vi "RT_Main.vi"() -> ()   [LabVIEW 2018]
uses:
  <vilib>/NI/STM/SubVIs/MetaDataElement.ctl
  RT_Listener_states.ctl
  RT_Counter_FGV_States.ctl
  RT_Comm_Manager_Message.ctl
  RT_Comm_Manager_States.ctl
  <vilib>/NI/STM/TCP/TCP Connection Info.ctl
  <vilib>/NI/STM/Connection Manager/TCP/TCP Connection Method.ctl
  <vilib>/NI/STM/TCP/TCP Write Options.ctl
  <vilib>/NI/STM/TCP/TCP Read Options.ctl
  <vilib>/NI/STM/TCP/Get Connection Reference (TCP).vi
  <vilib>/NI/STM/TCP/Read Meta Data (TCP Ref).vi
  <vilib>/NI/STM/SubVIs/Generate STM Error.vi
  <vilib>/NI/STM/TCP/Read Meta Data (TCP Clst).vi
  <vilib>/NI/STM/TCP/Read Message (TCP).vi
  <vilib>/NI/STM/TCP/Write Message (TCP).vi
  <vilib>/NI/STM/NI STM.lvlib
panel:
  out "Sensor not connected":bool
  out "meta data":T1[](array[typedef])
  in  "Max connections":i32=10
  out "Number of connections":i32
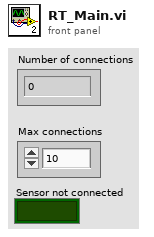
[diagram p1: front panel]
types:
  T1 = typedef "NI STM.lvlib/MetaDataElement.ctl" = string
  T2 = typedef "NI STM.lvlib/TCP Connection Info.ctl" = cluster{"connection ID":refnum<k5>, "meta data":T1[]}
  T3 = typedef "RT_Comm_Manager_Message.ctl" = cluster{"RT Comm Manager States":T4, "Data":variant}
  T4 = typedef "RT_Comm_Manager_States.ctl" = enum16{"Meas finished", "New connection", "Exit"}
  T5 = typedef "RT_Counter_FGV_States.ctl" = enum16{"Init", "Increase", "Decrease", "Get"}
  T6 = typedef "RT_Listener_states.ctl" = enum16{"Idle", "Listen", "Wait", "Exit"}
  T7 = typedef "NI STM.lvlib/TCP Connection Manager Reference.ctl" = refnum<data-value>
  T8 = typedef "NI STM.lvlib/TCP Read Options.ctl" = cluster{"ignore timeout error":bool, "timeout ms (1000)":i32}
  T9 = typedef "NI STM.lvlib/TCP Write Options.ctl" = cluster{"ignore timeout error":bool, "timeout ms (1000)":i32}
  T10 = typedef "NI STM.lvlib/TCP Connection Method.ctl" = enum16{"Initialize", "Add Connection", "Set Properties", "Get Connection(s)", "Remove Connection", "Remove All Connections", "Get Connection Count"}
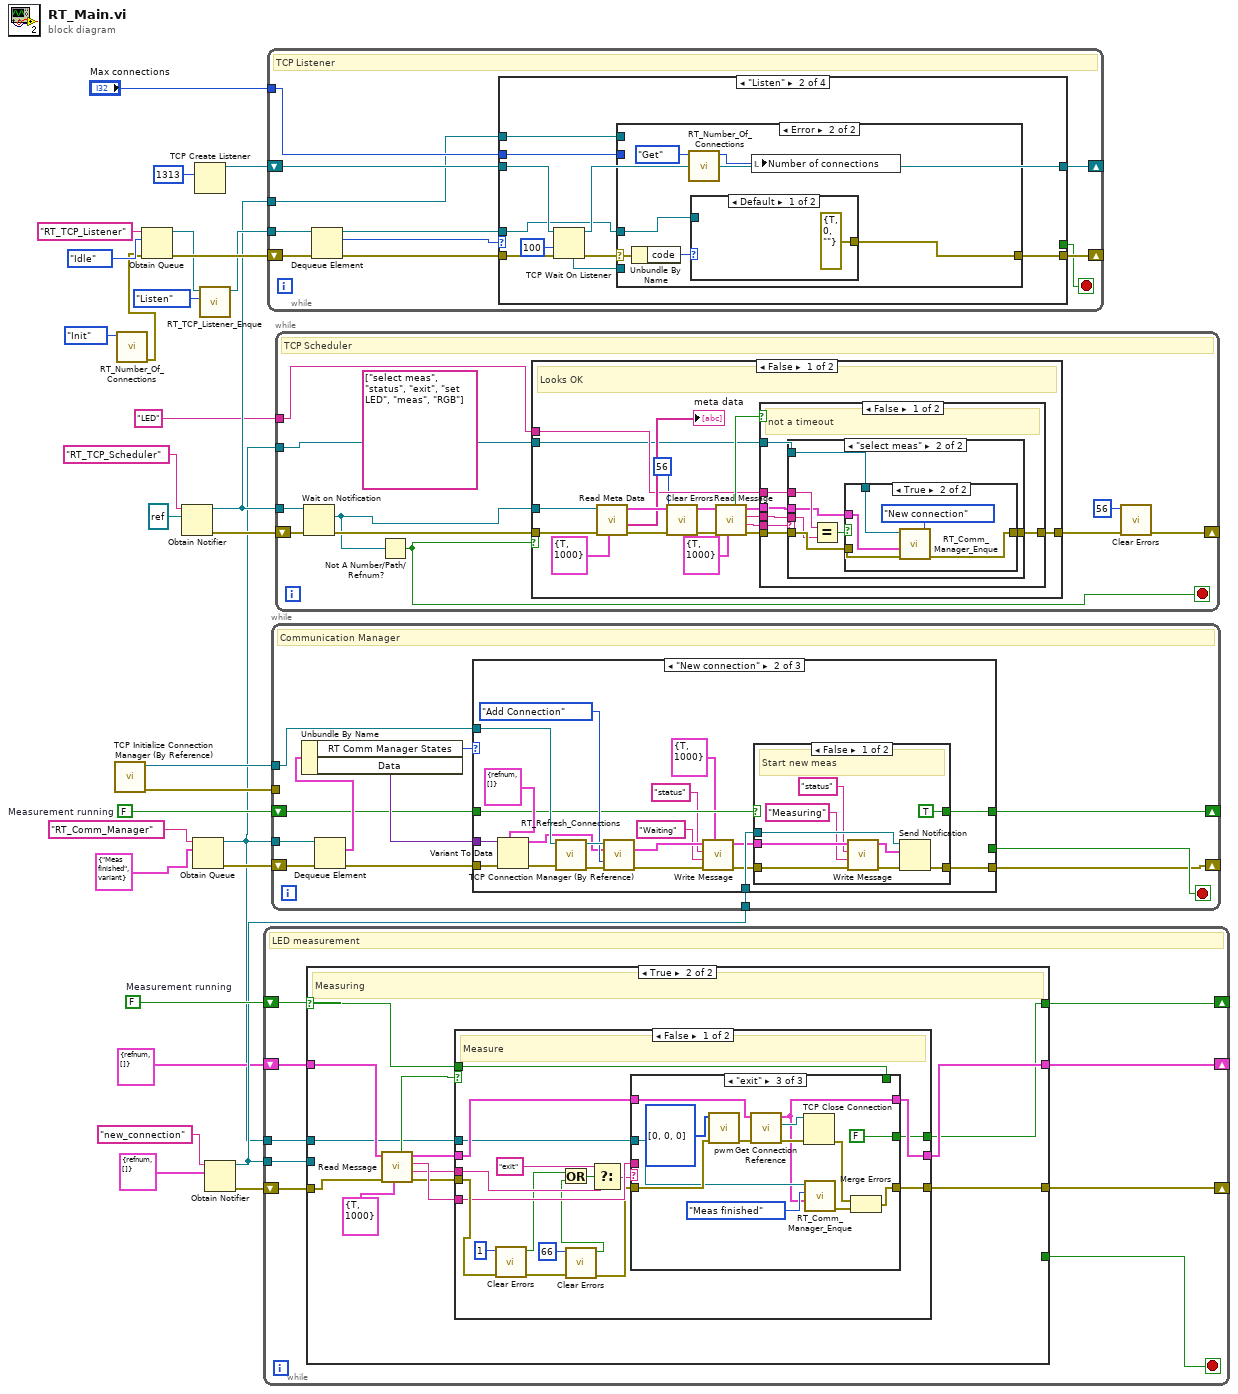
[diagram p0: block diagram]
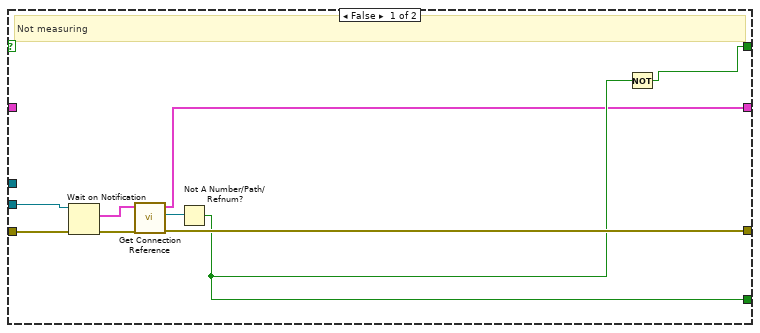
[diagram p2: hidden frame]
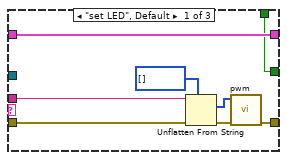
[diagram p3: hidden frame]
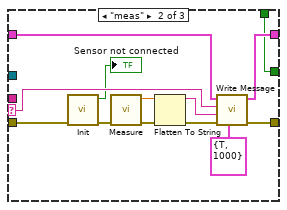
[diagram p4: hidden frame]
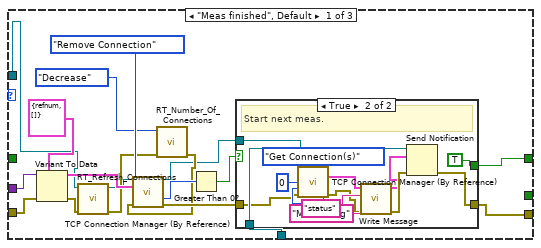
[diagram p6: hidden frame]
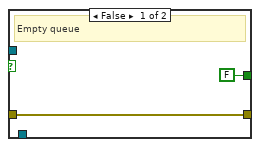
[diagram p7: hidden frame]
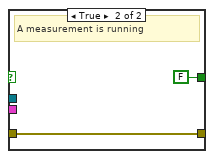
[diagram p8: hidden frame]
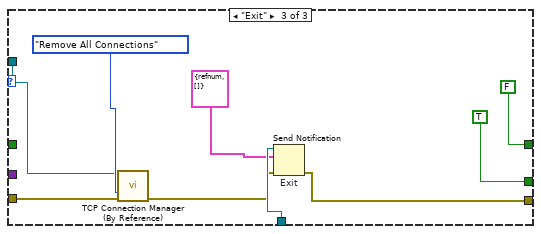
[diagram p9: hidden frame]
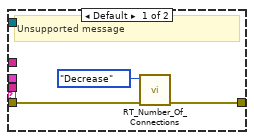
[diagram p10: hidden frame]
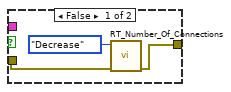
[diagram p11: hidden frame]
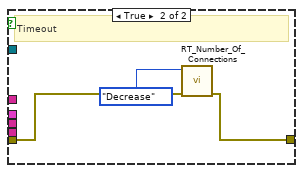
[diagram p12: hidden frame]
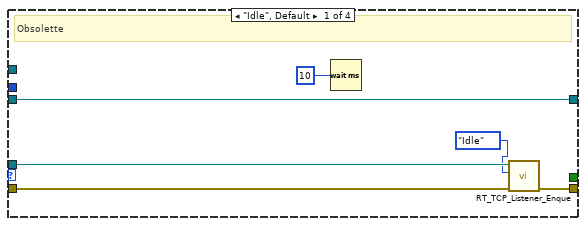
[diagram p14: hidden frame]
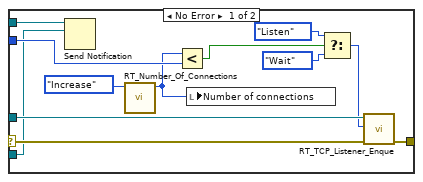
[diagram p15: hidden frame]
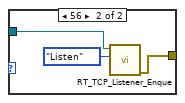
[diagram p16: hidden frame]
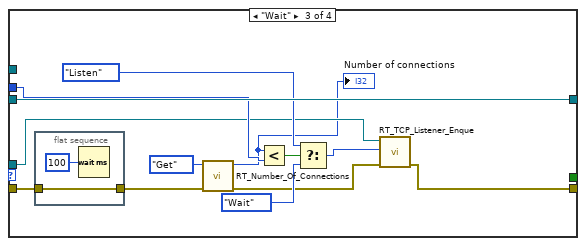
[diagram p17: hidden frame]
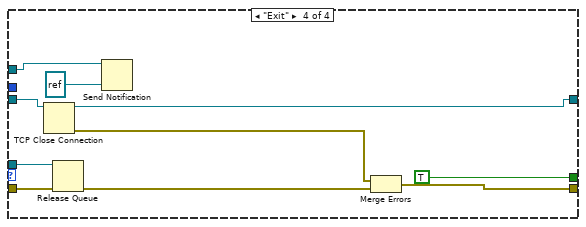
[diagram p18: hidden frame]
diagram:
  w7 = FALSE  # Measurement running
  w8 = FALSE  # Measurement running
  n1 = call <vilib>:"TCP Initialize Connection Manager (By Reference).vi"() -> ("error out"=w14:errorcluster, "connection manager ref out"=w13:T7)  [unwired: 10 in]
  n2 = call "RT_Number_Of_Connections.vi"("Counter_FGV_States"=RT_Counter_FGV_States."Init") -> ("Error Out"=w20:errorcluster)  [unwired: 9 in, 1 out]
  n3 = Obtain Queue(name (unnamed)="RT_TCP_Listener", element data type=RT_Listener_states."Idle" ("Listener States"), error in (no error)=w20) -> (queue out=w24:refnum<queue>, error out=w27:errorcluster)  [unwired: 2 in, 1 out]
  n4 = Obtain Notifier(name (unnamed)="RT_TCP_Scheduler", notification data type=refnum<k5> refnum ("connection ID")) -> (notifier out=w16:refnum<notifier>, error out=w15:errorcluster)  [unwired: 2 in, 1 out]
  n5 = Obtain Queue(name (unnamed)="RT_Comm_Manager", element data type=T3 {"RT Comm Manager States"=enum."Meas finished", "Data"=variant} ("Comm Manager Message")) -> (queue out=w1:refnum<queue>, error out=w9:errorcluster)  [unwired: 3 in, 1 out]
  n6 = TCP Create Listener(10:u16 1313 ("port")) -> (3:w25:refnum<k5>)  [unwired: 4 in, 2 out]
  n7 = call "RT_TCP_Listener_Enque.vi"("Listener States"=RT_Listener_states."Listen", "Queue In"=w24) -> ("Queue Out"=w23:refnum<queue>)  [unwired: 8 in, 1 out]
  n8 = Obtain Notifier(name (unnamed)="new_connection", notification data type=T2 {"connection ID"=refnum, "meta data"=[]} ("connection info out")) -> (notifier out=w3:refnum<notifier>, error out=w4:errorcluster)  [unwired: 2 in, 1 out]
  n9 = while {
    shift-right: [w37] -> _
    shift-left: w7 -> [w38]
    tunnel: w3 -> [w36]
    shift-right: [w33] -> _
    shift-left: w4 -> [w35]
    shift-right: [w32] -> _
    shift-left: T2 {"connection ID"=refnum, "meta data"=[]} ("connection info out") -> [w31]
    tunnel: w1 -> [w30]
    stop <- w34 stop-if-true
    # "LED measurement"
    n10 = case shown="True" w38 {
      selector: w38 -> [_ w48]
      tunnel: [w40 w49] -> w37
      tunnel: w36 -> [w47 _]
      tunnel: w35 -> [w46 w58]
      tunnel: [w41 _] -> w34
      tunnel: [w42 w60] -> w33
      tunnel: [w39 w54] -> w32
      tunnel: w31 -> [_ w57]
      tunnel: w30 -> [_ w51]
      frame False {
        # "Not measuring"
        n11 = Wait on Notification(notifier=w47, error in (no error)=w46) -> (notification=w44:T2, error out=w45:errorcluster)  [unwired: 2 in, 2 out]
        n12 = call-poly <vilib>:"Get Connection Reference.vi"("error in"=w45, "connection info in"=w44) -> ("error out"=w42:errorcluster, "connection ID out"=w43:refnum<k5>, "connection info out"=w39:T2)  [unwired: 7 in]
        n13 = Not A Number/Path/Refnum?(number/path/refnum=w43) -> (NaN/Path/Refnum?=w41:bool)
        n14 = Not(x=w41) -> (.not. x?=w40:bool)
      }
      frame True {
        # "Measuring"
        n15 = call-poly <vilib>:"Read Message.vi"("options"=T8 {"ignore timeout error"=TRUE, "timeout ms (1000)"=1000}, "error in"=w58, "connection info in"=w57) -> ("error out"=w50:errorcluster, "name"=w52:T1, "data string"=w53:string, "connection info out"=w55:T2, "timed out?"=w56:bool)  [unwired: 3 in, 1 out]
        n16 = case shown="False" w56 {
          tunnel: [w78 w114] -> w60
          tunnel: w50 -> [w77 w114]
          tunnel: w55 -> [w75 w115]
          tunnel: [w76 w115] -> w54
          tunnel: w53 -> [w74 _]
          tunnel: w52 -> [w71 _]
          tunnel: w51 -> [w73 _]
          tunnel: [w68 w113] -> w49
          tunnel: w48 -> [w67 w113]
          frame False {
            # "Measure"
            n17 = call <vilib>:"Clear Errors.vi"("error in (no error)"=w77, "specific error code to clear (0: all)"=1) -> ("error out"=w64:errorcluster, "specific error cleared?"=w70:bool)  [unwired: 4 in]
            n18 = call <vilib>:"Clear Errors.vi"("error in (no error)"=w64, "specific error code to clear (0: all)"=66) -> ("error out"=w63:errorcluster, "specific error cleared?"=w61:bool)  [unwired: 4 in]
            n19 = Or(x=w70, y=w61) -> (x .or. y?=w62:bool)
            n20 = Select(t=T1 "exit", s=w62, f=w71) -> (s? t:f=w72:T1)
            n21 = case shown="\"exit\"" w72 {
              selector: w72 -> [_ w96 _]
              tunnel: [w81 w98 w101] -> w76
              tunnel: [w83 w99 w104] -> w78
              tunnel: w63 -> [w82 w89 w108]
              tunnel: w75 -> [w81 w88 w107]
              tunnel: w74 -> [w80 _ _]
              tunnel: w73 -> [_ _ w103]
              tunnel: [w79 w87 FALSE] -> w68
              tunnel: w67 -> [w79 w87 _]
              frame "set LED", Default {
                n22 = Unflatten From String(type=u8[] [], binary string=w80, error in (no error)=w82) -> (value=w85:u8[], error out=w86:errorcluster)  [unwired: 2 in, 1 out]
                n23 = call "pwm.vi"("Error In"=w86, "PWMs"=w85) -> ("Error Out"=w83:errorcluster)  [unwired: 9 in]
              }
              frame "meas" {
                n24 = call "Init.vi"("Error In"=w89) -> ("Error Out"=w91:errorcluster, "Not connected"=→"Sensor not connected":bool)  [unwired: 9 in]
                n25 = call "Measure.vi"("Error In"=w91) -> ("Error Out"=w93:errorcluster, "Luminosity"=w92:dbl)  [unwired: 9 in]
                n26 = Flatten To String(anything=w92, error in (no error)=w93) -> (data string=w94:string, error out=w95:errorcluster)  [unwired: 2 in, 1 out]
                n27 = call-poly <vilib>:"Write Message.vi"("options"=T9 {"ignore timeout error"=TRUE, "timeout ms (1000)"=1000}, "error in"=w95, "data"=w94, "name"=w96, "connection info in"=w88) -> ("error out"=w99:errorcluster, "connection info out"=w98:T2)  [unwired: 5 in]
              }
              frame "exit" {
                n28 = call "pwm.vi"("Error In"=w108, "PWMs"=u8[] [0, 0, 0]) -> ("Error Out"=w110:errorcluster)  [unwired: 9 in]
                n29 = call-poly <vilib>:"Get Connection Reference.vi"("error in"=w110, "connection info in"=w107) -> ("error out"=w112:errorcluster, "connection ID out"=w111:refnum<k5>, "connection info out"=w101:T2)  [unwired: 7 in]
                n30 = TCP Close Connection(connection ID=w111, error in (no error)=w112) -> (error out=w105:errorcluster)  [unwired: 1 in, 1 out]
                n31 = call "RT_Comm_Manager_Enque.vi"("Data"=w101, "Next State"=RT_Comm_Manager_States."Meas finished", "Queue In"=w103) -> ("Error Out"=w106:errorcluster)  [unwired: 7 in, 1 out]
                n32 = Merge Errors(w105, w106) -> (w104:errorcluster)
              }
            }
          }
          frame True {
            # "Timeout"
          }
        }
      }
    }
  }
  n33 = while {
    tunnel: w23 -> [w126]
    shift-right: [w121] -> _
    shift-left: w27 -> [w125]
    shift-right: [w118] -> _
    shift-left: w25 -> [w119]
    tunnel: "Max connections" -> [w117]
    tunnel: w16 -> [w116]
    stop <- w120 stop-if-true
    # "TCP Listener"
    n34 = Dequeue Element(queue=w126, error in (no error)=w125) -> (queue out=w122:refnum<queue>, element=w123:T6, error out=w124:errorcluster)  [unwired: 1 in, 1 out]
    n35 = case shown="\"Listen\"" w123 {
      tunnel: w124 -> [w131 w142 w174 w189]
      tunnel: w122 -> [w129 w138 w166 w186]
      tunnel: [w130 w137 w168 w184] -> w121
      tunnel: [_ _ _ TRUE] -> w120
      tunnel: w119 -> [w132 w141 w177 w185]
      tunnel: [w132 w140 w177 w182] -> w118
      tunnel: w117 -> [_ w134 w173 _]
      tunnel: w116 -> [_ w133 _ w181]
      frame "Idle", Default {
        # "Obsolette"
        n36 = Wait (ms)(milliseconds to wait=u32 10) -> ()  [unwired: 1 out]
        n37 = call "RT_TCP_Listener_Enque.vi"("Error In"=w131, "Listener States"=RT_Listener_states."Idle", "Queue In"=w129) -> ("Error Out"=w130:errorcluster)  [unwired: 7 in, 1 out]
      }
      frame "Listen" {
        n38 = TCP Wait On Listener(8:w142, 9:100 ("timeout ms (wait forever: -1)"), 11:w141) -> (0:w136:errorcluster, 3:w140:refnum<k5>, 4:w135:refnum<k5>)  [unwired: 1 in, 2 out]
        n39 = case shown="Error" w136 {
          selector: w136 -> [w152 w160]
          tunnel: w138 -> [w154 w158]
          tunnel: [w153 w157] -> w137
          tunnel: w135 -> [w144 _]
          tunnel: w134 -> [w150 _]
          tunnel: w133 -> [w145 _]
          frame No Error {
            n40 = Send Notification(notification=w144, notifier=w145) -> ()  [unwired: 1 in, 2 out]
            n41 = call "RT_Number_Of_Connections.vi"("Counter_FGV_States"=RT_Counter_FGV_States."Increase") -> ("Number of connections"=w143:i32)  [unwired: 9 in, 1 out]
            n42 = Less?(x=w143, y=w150) -> (x < y?=w149:bool)
            n43 = local write "Number of connections"(w143) -> ()
            n44 = Select(t=RT_Listener_states."Listen" ("Listener States"), s=w149, f=RT_Listener_states."Wait") -> (s? t:f=w146:T6)
            n45 = call "RT_TCP_Listener_Enque.vi"("Error In"=w152, "Listener States"=w146, "Queue In"=w154) -> ("Error Out"=w153:errorcluster)  [unwired: 7 in, 1 out]
          }
          frame Error {
            n46 = Unbundle By Name(w160) -> ("code"=w159:i32)
            n47 = call "RT_Number_Of_Connections.vi"("Counter_FGV_States"=RT_Counter_FGV_States."Get") -> ("Number of connections"=w155:i32)  [unwired: 9 in, 1 out]
            n48 = case shown="Default" w159 {
              tunnel: w158 -> [_ w164]
              tunnel: [errorcluster {"status"=TRUE, "code"=0, "source"=""} ("Error Out") w162] -> w157
              frame Default {
              }
              frame 56 {
                n49 = call "RT_TCP_Listener_Enque.vi"("Listener States"=RT_Listener_states."Listen", "Queue In"=w164) -> ("Error Out"=w162:errorcluster)  [unwired: 8 in, 1 out]
              }
            }
            n50 = local write "Number of connections"(w155) -> ()
          }
        }
      }
      frame "Wait" {
        n51 = flat-sequence {
          tunnel: [w178] -> w175
          tunnel: w174 -> [w178]
          frame #0 {
            n52 = Wait (ms)(milliseconds to wait=u32 100) -> ()  [unwired: 1 out]
          }
        }
        n53 = call "RT_Number_Of_Connections.vi"("Error In"=w175, "Counter_FGV_States"=RT_Counter_FGV_States."Get") -> ("Error Out"=w169:errorcluster, "Number of connections"=w165:i32)  [unwired: 8 in]
        "Number of connections" <- w165
        n54 = Less?(x=w165, y=w173) -> (x < y?=w172:bool)
        n55 = Select(t=RT_Listener_states."Listen" ("Listener States"), s=w172, f=RT_Listener_states."Wait" ("Listener States")) -> (s? t:f=w167:T6)
        n56 = call "RT_TCP_Listener_Enque.vi"("Error In"=w169, "Listener States"=w167, "Queue In"=w166) -> ("Error Out"=w168:errorcluster)  [unwired: 7 in, 1 out]
      }
      frame "Exit" {
        n57 = TCP Close Connection(connection ID=w185) -> (connection ID out=w182:refnum<k5>, error out=w183:errorcluster)  [unwired: 2 in]
        n58 = Release Queue(queue=w186, error in (no error)=w189) -> (error out=w188:errorcluster)  [unwired: 1 in, 2 out]
        n59 = Send Notification(notification=refnum<k5> refnum ("connection ID"), notifier=w181) -> ()  [unwired: 1 in, 2 out]
        n60 = Merge Errors(w183, w188) -> (w184:errorcluster)
      }
    }
  }
  n61 = while {
    tunnel: w14 -> [_]
    tunnel: w13 -> [w195]
    tunnel: w1 -> [w201]
    shift-right: [w193] -> _
    shift-left: w9 -> [w200]
    shift-right: [w191] -> _
    shift-left: w8 -> [w192]
    tunnel: w3 -> [w190]
    stop <- w194 stop-if-true
    # "Communication Manager"
    n62 = Dequeue Element(queue=w201, error in (no error)=w200) -> (element=w199:T3, error out=w197:errorcluster)  [unwired: 1 in, 2 out]
    n63 = Unbundle By Name(w199) -> ("RT Comm Manager States"=w198:T4, "Data"=w196:variant)
    n64 = case shown="\"New connection\"" w198 {
      tunnel: w197 -> [w217 w254 w274]
      tunnel: w196 -> [w215 w253 _]
      tunnel: w195 -> [w207 w250 w270]
      tunnel: [w209 w244 w266] -> w193
      tunnel: [_ _ TRUE] -> w194
      tunnel: w192 -> [_ w245 _]
      tunnel: [w210 w243 FALSE] -> w191
      tunnel: w190 -> [w208 w242 w269]
      frame "Meas finished", Default {
        n65 = Variant To Data(error in=w217, type=T2 {"connection ID"=refnum, "meta data"=[]} ("connection info out"), Variant=w215) -> (data=w214:T2, error out=w216:errorcluster)
        n66 = call "RT_Refresh_Connections.vi"("Error In"=w216, "connection manager ref in"=w207) -> ("Error Out"=w204:errorcluster, "connection manager ref out"=w206:T7)  [unwired: 8 in]
        n67 = call "RT_Number_Of_Connections.vi"("Error In"=w204, "Counter_FGV_States"=RT_Counter_FGV_States."Decrease") -> ("Error Out"=w203:errorcluster)  [unwired: 8 in, 1 out]
        n68 = call <vilib>:"TCP Connection Manager (By Reference).vi"("connection manager ref in"=w206, "connection in"=w214, "method"=TCP_Connection_Method."Remove Connection", "error in"=w203) -> ("connection manager ref out"=w202:T7, "number of connections"=w213:i32, "error out"=w212:errorcluster)  [unwired: 5 in, 4 out]
        n69 = Greater Than 0?(x=w213) -> (x > 0?=w211:bool)
        n70 = case shown="True" w211 {
          tunnel: w212 -> [w221 w228]
          tunnel: [FALSE TRUE] -> w210
          tunnel: [w221 w232] -> w209
          tunnel: w208 -> [_ w233]
          tunnel: w202 -> [_ w229]
          frame False {
            # "Empty queue"
          }
          frame True {
            # "Start next meas."
            n71 = call <vilib>:"TCP Connection Manager (By Reference).vi"("connection manager ref in"=w229, "index"=0, "method"=TCP_Connection_Method."Get Connection(s)", "error in"=w228) -> ("connection out"=w227:T2, "error out"=w223:errorcluster)  [unwired: 5 in, 5 out]
            n72 = call-poly <vilib>:"Write Message.vi"("error in"=w223, "data"="Measuring", "name"="status", "connection info in"=w227) -> ("error out"=w224:errorcluster, "connection info out"=w222:T2)  [unwired: 6 in]
            n73 = Send Notification(notification=w222, notifier=w233, error in (no error)=w224) -> (error out=w232:errorcluster)  [unwired: 1 out]
          }
        }
      }
      frame "New connection" {
        n74 = Variant To Data(error in=w254, type=T2 {"connection ID"=refnum, "meta data"=[]} ("connection info out"), Variant=w253) -> (data=w246:T2, error out=w251:errorcluster)
        n75 = call "RT_Refresh_Connections.vi"("Error In"=w251, "connection manager ref in"=w250) -> ("Error Out"=w247:errorcluster, "connection manager ref out"=w249:T7)  [unwired: 8 in]
        n76 = call <vilib>:"TCP Connection Manager (By Reference).vi"("connection manager ref in"=w249, "connection in"=w246, "method"=TCP_Connection_Method."Add Connection", "error in"=w247) -> ("connection out"=w241:T2, "error out"=w239:errorcluster)  [unwired: 5 in, 5 out]
        n77 = call-poly <vilib>:"Write Message.vi"("options"=T9 {"ignore timeout error"=TRUE, "timeout ms (1000)"=1000}, "error in"=w239, "data"="Waiting", "name"="status", "connection info in"=w241) -> ("error out"=w238:errorcluster, "connection info out"=w240:T2)  [unwired: 5 in]
        n78 = case shown="False" w245 {
          tunnel: w238 -> [w259 w265]
          tunnel: [w261 w265] -> w244
          tunnel: [TRUE FALSE] -> w243
          tunnel: w240 -> [w260 _]
          tunnel: w242 -> [w262 _]
          frame False {
            # "Start new meas"
            n79 = call-poly <vilib>:"Write Message.vi"("error in"=w259, "data"="Measuring", "name"="status", "connection info in"=w260) -> ("error out"=w257:errorcluster, "connection info out"=w258:T2)  [unwired: 6 in]
            n80 = Send Notification(notification=w258, notifier=w262, error in (no error)=w257) -> (error out=w261:errorcluster)  [unwired: 1 out]
          }
          frame True {
            # "A measurement is running"
          }
        }
      }
      frame "Exit" {
        n81 = call <vilib>:"TCP Connection Manager (By Reference).vi"("connection manager ref in"=w270, "method"=TCP_Connection_Method."Remove All Connections", "error in"=w274) -> ("error out"=w267:errorcluster)  [unwired: 6 in, 6 out]
        n82 = Send Notification "Exit"(notification=T2 {"connection ID"=refnum, "meta data"=[]}, notifier=w269, error in (no error)=w267) -> (error out=w266:errorcluster)  [unwired: 1 out]
      }
    }
  }
  n83 = while {
    tunnel: w16 -> [w284]
    shift-right: [w276] -> _
    shift-left: w15 -> [w283]
    tunnel: "LED" -> [w278]
    tunnel: w1 -> [w277]
    stop <- w280 stop-if-true
    (unwired) T1[] ["select meas", "status", "exit", "set LED", "meas", "RGB"] ("meta data")
    # "TCP Scheduler"
    n84 = Wait on Notification(notifier=w284, error in (no error)=w283) -> (notification=w281:refnum<k5>, error out=w282:errorcluster)  [unwired: 2 in, 2 out]
    n85 = Not A Number/Path/Refnum?(number/path/refnum=w281) -> (NaN/Path/Refnum?=w280:bool)
    n86 = case shown="False" w280 {
      tunnel: w282 -> [w301 w330]
      tunnel: w281 -> [w300 _]
      tunnel: [w289 w330] -> w279
      tunnel: w278 -> [w288 _]
      tunnel: w277 -> [w287 _]
      frame False {
        # "Looks OK"
        n87 = call-poly <vilib>:"Read Meta Data.vi"("options"=T8 {"ignore timeout error"=TRUE, "timeout ms (1000)"=1000}, "error in"=w301, "connection ID"=w300) -> ("error out"=w298:errorcluster, "meta data"=→"meta data":T1[], "connection info out"=w297:T2)  [unwired: 6 in]
        n88 = call <vilib>:"Clear Errors.vi"("error in (no error)"=w298, "specific error code to clear (0: all)"=56) -> ("error out"=w286:errorcluster)  [unwired: 4 in, 1 out]
        n89 = call-poly <vilib>:"Read Message.vi"("options"=T8 {"ignore timeout error"=TRUE, "timeout ms (1000)"=1000}, "error in"=w286, "connection info in"=w297) -> ("error out"=w294:errorcluster, "name"=w292:T1, "data string"=w290:string, "connection info out"=w291:T2, "timed out?"=w293:bool)  [unwired: 3 in, 1 out]
        n90 = case shown="False" w293 {
          tunnel: w294 -> [w308 w329]
          tunnel: w292 -> [w307 _]
          tunnel: w291 -> [w306 _]
          tunnel: w290 -> [w305 _]
          tunnel: [w304 w328] -> w289
          tunnel: w288 -> [w303 _]
          tunnel: w287 -> [w302 _]
          frame False {
            # "not a timeout"
            n91 = case shown="\"select meas\"" w307 {
              tunnel: w308 -> [w310 w318]
              tunnel: w306 -> [_ w312]
              tunnel: w305 -> [_ w316]
              tunnel: [w309 w317] -> w304
              tunnel: w303 -> [_ w315]
              tunnel: w302 -> [_ w313]
              frame Default {
                # "Unsupported message"
                n92 = call "RT_Number_Of_Connections.vi"("Error In"=w310, "Counter_FGV_States"=RT_Counter_FGV_States."Decrease") -> ("Error Out"=w309:errorcluster)  [unwired: 8 in, 1 out]
              }
              frame "select meas" {
                n93 = Equal?(x=w315, y=w316) -> (x = y?=w314:bool)
                n94 = case shown="True" w314 {
                  tunnel: w318 -> [w320 w326]
                  tunnel: [w319 w323] -> w317
                  tunnel: w313 -> [_ w325]
                  tunnel: w312 -> [_ w322]
                  frame False {
                    n95 = call "RT_Number_Of_Connections.vi"("Error In"=w320, "Counter_FGV_States"=RT_Counter_FGV_States."Decrease") -> ("Error Out"=w319:errorcluster)  [unwired: 8 in, 1 out]
                  }
                  frame True {
                    n96 = call "RT_Comm_Manager_Enque.vi"("Error In"=w326, "Data"=w322, "Next State"=RT_Comm_Manager_States."New connection", "Queue In"=w325) -> ("Error Out"=w323:errorcluster)  [unwired: 6 in, 1 out]
                  }
                }
              }
            }
          }
          frame True {
            # "Timeout"
            n97 = call "RT_Number_Of_Connections.vi"("Error In"=w329, "Counter_FGV_States"=RT_Counter_FGV_States."Decrease") -> ("Error Out"=w328:errorcluster)  [unwired: 8 in, 1 out]
          }
        }
      }
      frame True {
        # "Not a refnum"
      }
    }
    n98 = call <vilib>:"Clear Errors.vi"("error in (no error)"=w279, "specific error code to clear (0: all)"=56) -> ("error out"=w276:errorcluster)  [unwired: 4 in, 1 out]
  }
